vi "pb_stop.vi"(8 "error in (no error)":errorcluster, 11 "path in":path=path "C:/Program Files/SpinCore/SpinAPI/dll/spinapi.dll") -> (0 "error out":errorcluster, 3 "path out":path)   [LabVIEW 2016]
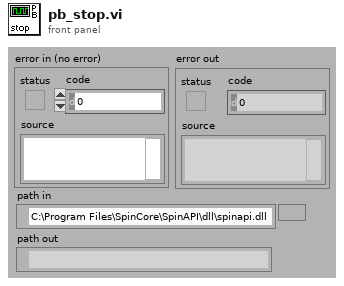
[diagram p1: front panel]
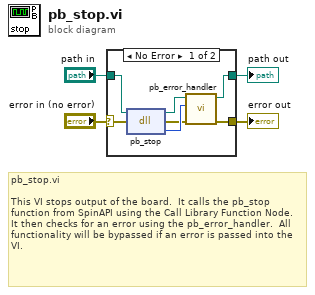
[diagram p0: block diagram]
diagram:
  # "pb_stop.vi\n\nThis VI stops output of the board.  It calls the pb_stop function from SpinAPI using the Call Library Function Node.  It then checks for an error using the pb_error_handler.  All functionality will be bypassed if an error is passed into the VI."
  n1 = case shown="No Error" "error in (no error)" {
    selector: "error in (no error)" -> [w10 w13]
    tunnel: [w6 w13] -> w4
    tunnel: "path in" -> [w9 w12]
    tunnel: [w5 w12] -> w1
    frame No Error {
      n2 = dll-call lib="C:/Program Files/SpinCore/SpinAPI/dll/spinapi.dll" fn="pb_stop"(path in=w9, error in=w10) -> (path out=w8:path, error out=w7:errorcluster, "return type"=w11:i32)  [unwired: 1 in]
      n3 = call "pb_error_handler.vi"("error in (no error)"=w7, "return code"=w11, "path in"=w8) -> ("error out"=w6:errorcluster, "path out"=w5:path)  [unwired: 7 out]
    }
    frame Error {
    }
  }
  "error out" <- w4
  "path out" <- w1
